vi "Toggle Vortex Direction.vi"(0 "Notifier Name":string, 11 "Error In":errorcluster) -> (4 "Notifier Name Dup":string, 8 "SLM Status":T1, 15 "Error Out":errorcluster)   [LabVIEW 2018]
uses:
  Hamamatsu/X10468 Series/X10468 Controls/X10468 SLM Notifier.ctl
  Hamamatsu/X10468 Series/X10468 Controls/X10468 SLM Actions.ctl
  <vilib>/vision/Image Controls.llb/IMAQ Image.ctl
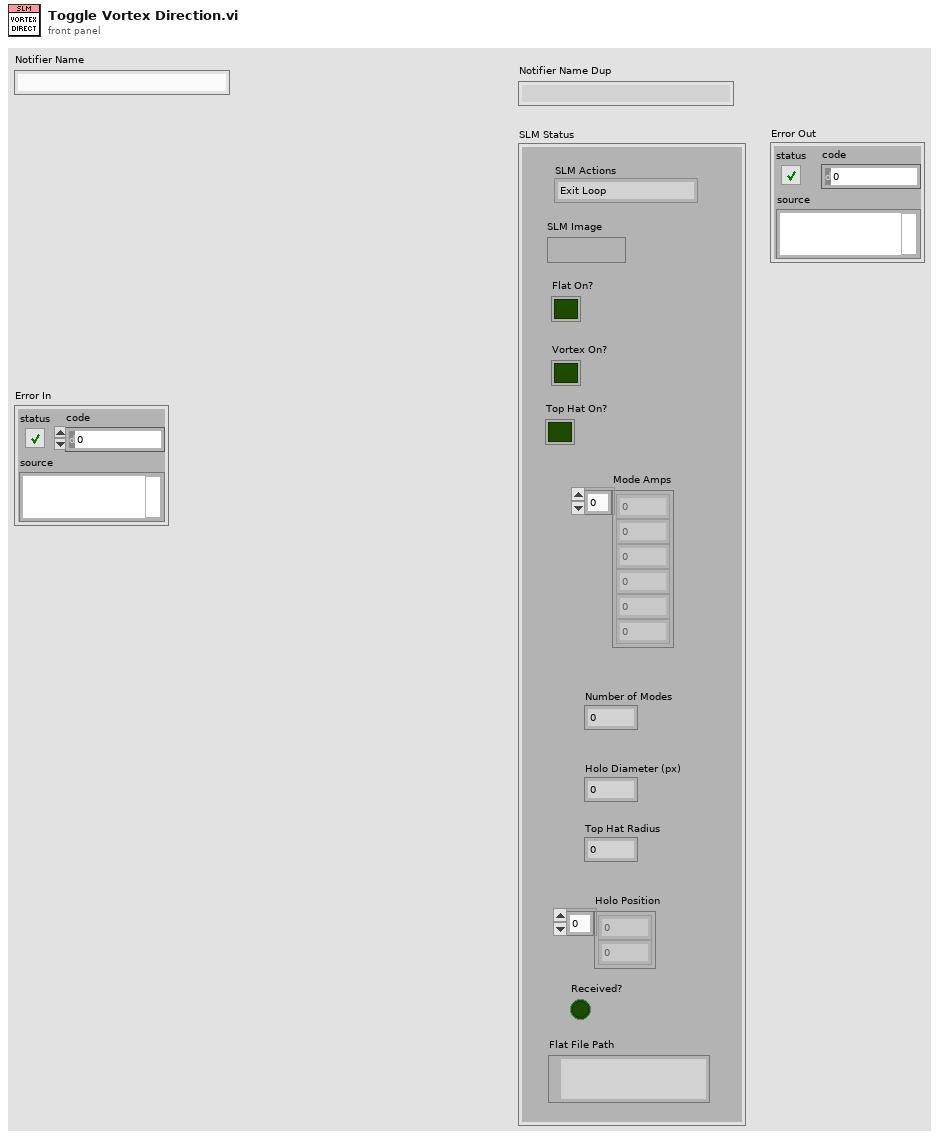
[diagram p1: front panel]
types:
  T1 = typedef "X10468 SLM Notifier.ctl" = cluster{"SLM Actions":T2, "SLM Image":T3, "Flat On?":bool, "Vortex On?":bool, "Top Hat On?":bool, "Mode Amps":dbl[], "Number of Modes":i32, "Holo Diameter (px)":i32, "Top Hat Radius":dbl, "Holo Position":i32[], "Received?":bool, "Flat File Path":path}
  T2 = typedef "X10468 SLM Actions.ctl" = enum16{"Exit Loop", "Get Settings", "Set Flat File", "Change Holo Size", "Change Num Modes", "Change Holo Position", "Change Top Hat Size", "Change Vortex Direction", "Change Mode Amounts", "Flat On/Off", "Vortex On/Off", "Top Hat On/Off", "Make Hologram", "Update SLM Display", "Quit"}
  T3 = typedef "IMAQ Image.ctl" = refnum<image>
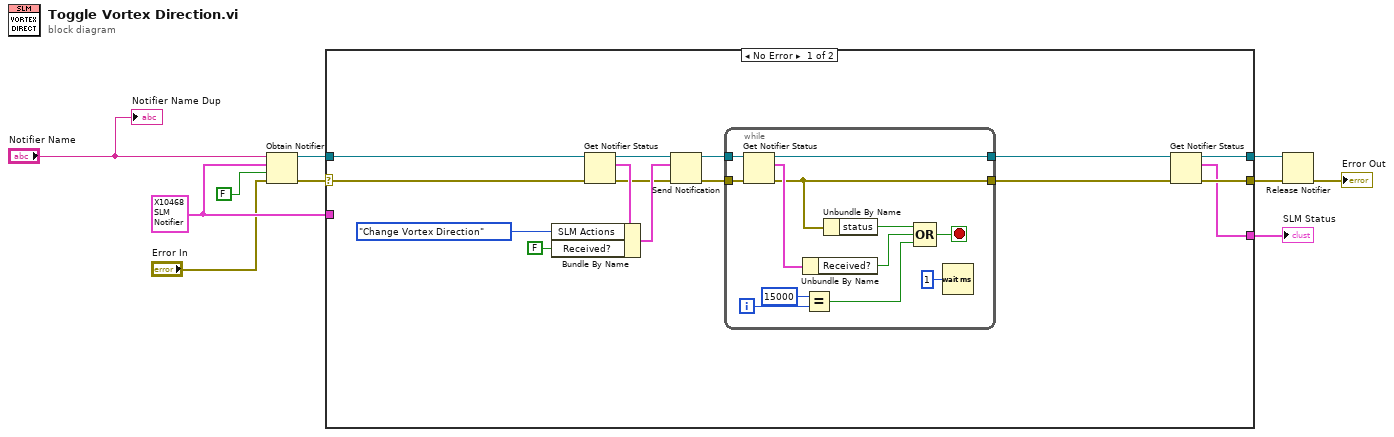
[diagram p0: block diagram]
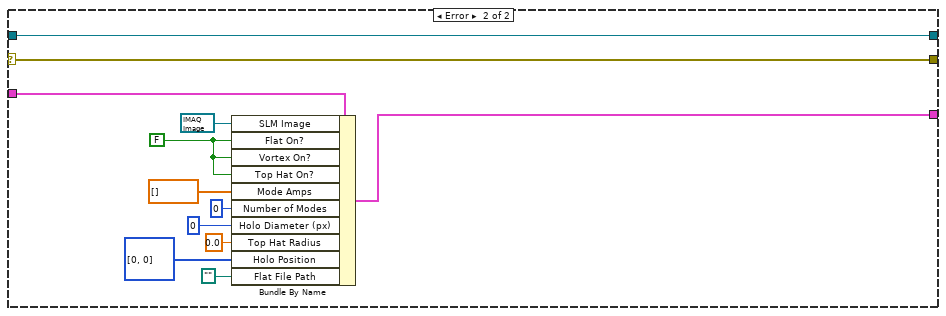
[diagram p2: hidden frame]
diagram:
  w2 = T1 {"SLM Actions"=enum."Exit Loop", "SLM Image"=refnum, "Flat On?"=FALSE, "Vortex On?"=FALSE, "Top Hat On?"=FALSE, "Mode Amps"=[], "Number of Modes"=0, "Holo Diameter (px)"=0, "Top Hat Radius"=0.0, "Holo Position"=[], "Received?"=FALSE, "Flat File Path"=path ""} ("SLM Notifier")
  n1 = Obtain Notifier(name (unnamed)="Notifier Name", notification data type=w2, create if not found? (T)=FALSE, error in (no error)="Error In") -> (notifier out=w8:refnum<notifier>, error out=w7:errorcluster)  [unwired: 1 out]
  n2 = case shown="No Error" w7 {
    selector: w7 -> [w23 w48]
    tunnel: w8 -> [w24 w49]
    tunnel: [w20 w49] -> w6
    tunnel: [w19 w48] -> w5
    tunnel: [w18 w46] -> w3
    tunnel: w2 -> [_ w47]
    frame No Error {
      n3 = Get Notifier Status(notifier=w24, error in (no error)=w23) -> (notifier out=w17:refnum<notifier>, current notification=w16:T1, error out=w14:errorcluster)  [unwired: 2 out]
      n4 = Bundle By Name(cluster=w16, "SLM Actions"=X10468_SLM_Actions."Change Vortex Direction", "Received?"=FALSE) -> (w15:T1)
      n5 = Send Notification(notification=w15, notifier=w17, error in (no error)=w14) -> (notifier out=w12:refnum<notifier>, error out=w11:errorcluster)
      n6 = while {
        tunnel: w12 -> [w37]
        tunnel: [w34] -> w22
        tunnel: w11 -> [w31]
        tunnel: [w30] -> w21
        i -> [w33]
        stop <- w26 stop-if-true
        n7 = Get Notifier Status(notifier=w37, error in (no error)=w31) -> (notifier out=w34:refnum<notifier>, current notification=w36:T1, error out=w30:errorcluster)  [unwired: 2 out]
        n8 = Unbundle By Name(w36) -> ("Received?"=w28:bool)
        n9 = Equal?(x=15000, y=w33) -> (x = y?=w27:bool)
        n10 = Unbundle By Name(w30) -> ("status"=w29:bool)
        n11 = Compound Arithmetic op=OR(w29, w28, w27) -> (w26:bool)
        n12 = Wait (ms)(milliseconds to wait=u32 1) -> ()  [unwired: 1 out]
      }
      n13 = Get Notifier Status(notifier=w22, error in (no error)=w21) -> (notifier out=w20:refnum<notifier>, current notification=w18:T1, error out=w19:errorcluster)  [unwired: 2 out]
    }
    frame Error {
      w44 = FALSE ("Flat On?")
      n14 = Bundle By Name(cluster=w47, "SLM Image"=T3 refnum, "Flat On?"=w44, "Vortex On?"=w44, "Top Hat On?"=w44, "Mode Amps"=dbl[] [], "Number of Modes"=0, "Holo Diameter (px)"=0, "Top Hat Radius"=0.0, "Holo Position"=i32[] [0, 0], "Flat File Path"=path "") -> (w46:T1)
    }
  }
  "SLM Status" <- w3
  n15 = Release Notifier(notifier=w6, error in (no error)=w5) -> (error out=→"Error Out":errorcluster)  [unwired: 1 in, 2 out]
  "Notifier Name Dup" <- "Notifier Name"
